vi "Initialization Module.vi"(8 "error in (no error)":errorcluster, 11 "Axis Resources In":refnum<k21>[](array[refnum])) -> (0 "error out":errorcluster, 3 "Axis Resources Out":refnum<k21>[](array[refnum]))   [LabVIEW 2014]
uses:
  <vilib>/Motion/Express/_s/nimc.ex.clearFaults.clearFaults.axis.vi
  <vilib>/Motion/Express/_s/nimc.ex.power.power.axis.vi
  <vilib>/Motion/Express/_s/nimc.ex.resetPosition.resetPosition.axis.vi
  <vilib>/Motion/BlockNode/FB.NIMotion.xnode
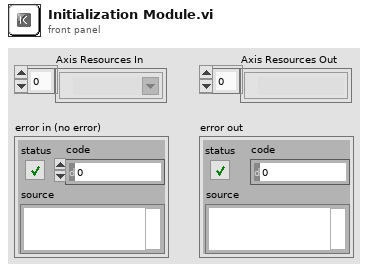
[diagram p1: front panel]
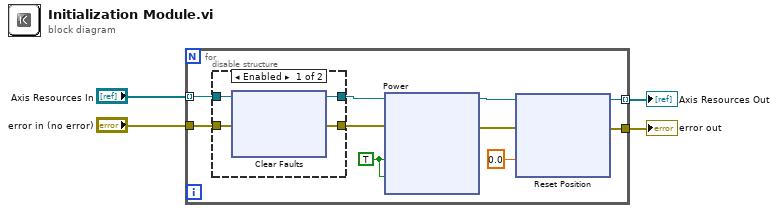
[diagram p0: block diagram]
diagram:
  n1 = for {
    tunnel: "Axis Resources In" -> [w14] mode=indexing
    tunnel: "error in (no error)" -> [w13]
    tunnel: [w12] -> w4
    tunnel: [w5] -> w3 mode=indexing
    w7 = TRUE ("enable axis")
    n2 = disable-structure shown="Enabled" {
      disable-tunnel: w14 -> [w18 w24]
      disable-tunnel: w13 -> [w17 w23]
      disable-tunnel: [w16 w24] -> w10
      disable-tunnel: [w15 w23] -> w8
      frame Enabled {
        n3 = xnode ("Clear Faults")("resource"=w18, "error in"=w17) -> ("resource out"=w16:refnum<k21>, "error out"=w15:errorcluster)
      }
      frame Disabled {
      }
    }
    n4 = xnode ("Power")("enable axis"=w7, "enable drive"=w7, "resource"=w10, "error in"=w8) -> ("resource out"=w9:refnum<k21>, "error out"=w6:errorcluster)
    n5 = xnode ("Reset Position")("position"=0.0, "resource"=w9, "error in"=w6) -> ("resource out"=w5:refnum<k21>, "error out"=w12:errorcluster)
  }
  "error out" <- w4
  "Axis Resources Out" <- w3
